vi "Analyse Board.vi"(8 "error in (no error)":errorcluster, 10 "GameBoard":u8[][](array[numeric]), 11 "CS++GoBangServer in":refnum<class "CS++GoBangServer.lvclass">) -> (0 "error out":errorcluster, 3 "CS++GoBangServer out":refnum<class "CS++GoBangServer.lvclass">)   [LabVIEW 2014, in "GoBang.lvlib" / "CS++GoBangServer.lvclass"]
uses:
  CS++GoBangServer.lvclass
  typdefs/GameState.ctl
  CS++GoBangServer.lvclass/CS++GoBangServer.ctl
  CSPP_Core/Classes/CS++ProcessVariables/ProcessVariable/PV.lvclass/PV.ctl
  CSPP_Core/Classes/CS++ProcessVariables/ProcessVariable/Write Data.vi
  GoBang.lvlib
  CSPP_Core/Classes/CS++ProcessVariables/ProcessVariable/PV.lvclass
  CSPP_Core/Classes/CS++ProcessVariables/PVConnection/PVConnection.lvclass
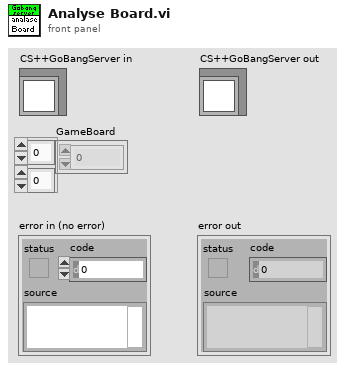
[diagram p1: front panel]
types:
  T1 = typedef "GoBang.lvlib/GameState.ctl" = enum16{"Waiting for opponent", "White to move", "Black to move", "Game over, white won", "Game over, black won"}
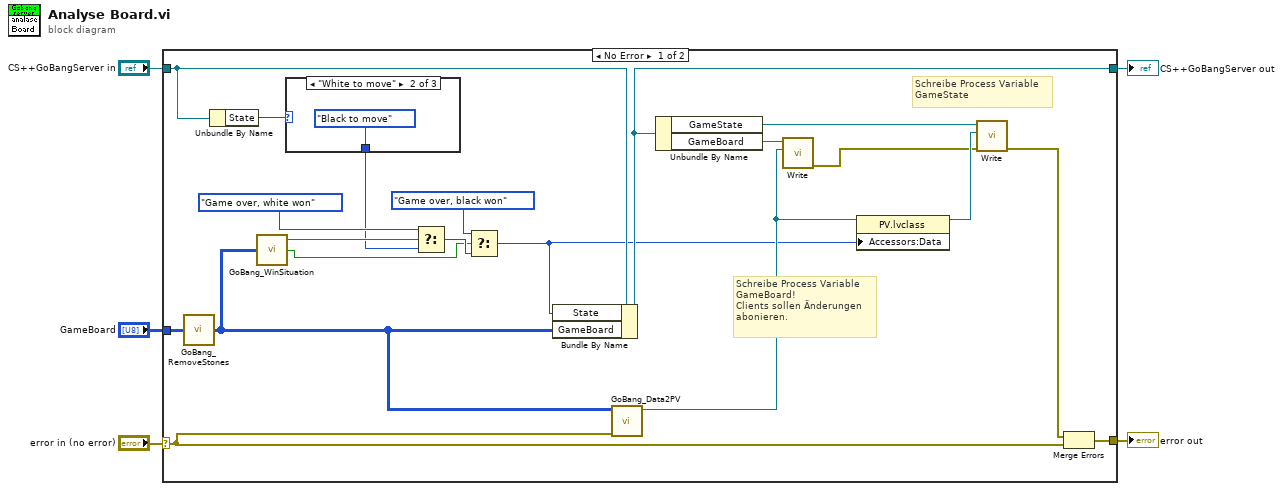
[diagram p0: block diagram]
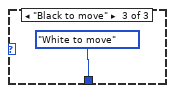
[diagram p3: hidden frame]
diagram:
  n1 = case shown="No Error" "error in (no error)" {
    selector: "error in (no error)" -> [w22 w30]
    tunnel: [w20 w30] -> w4
    tunnel: [w24 w29] -> w2
    tunnel: "CS++GoBangServer in" -> [w13 w29]
    tunnel: "GameBoard" -> [w25 _]
    frame No Error {
      # "Schreibe Process Variable \nGameState"
      # "Schreibe Process Variable \nGameBoard!\nClients sollen Änderungen\nabonieren."
      n2 = call "GoBang_RemoveStones.vi"("GameBoard in"=w25) -> ("GameBoard out"=w21:u8[][])
      n3 = Unbundle By Name(w13) -> ("State"=w9:T1)
      n4 = call "GoBang_WinSituation.vi"("GameBoard"=w21) -> ("White won"=w15:bool, "Black won"=w11:bool)  [unwired: 1 out]
      n5 = case shown="\"White to move\"" w9 {
        selector: w9 -> [w26 _ _]
        tunnel: [w26 GameState."Black to move" ("State") GameState."White to move" ("State")] -> w8
        frame "Waiting for opponent", Default {
        }
        frame "White to move" {
        }
        frame "Black to move" {
        }
      }
      n6 = Select(t=GameState."Game over, white won" ("State"), s=w15, f=w8) -> (s? t:f=w12:T1)
      n7 = Select(t=GameState."Game over, black won" ("State"), s=w11, f=w12) -> (s? t:f=w7:T1)
      n8 = Bundle By Name(cluster=w13, "State"=w7, "GameBoard"=w21) -> (w24:refnum<class "CS++GoBangServer.lvclass">)
      n9 = call "GoBang_Data2PV.vi"("error in (no error)"=w22, "Data in"=w21) -> ("PV out"=w18:refnum<class "PV.lvclass">)  [unwired: 9 in]
      n10 = Unbundle By Name(w24) -> ("GameState"=w19:refnum<class "PVConnection.lvclass">, "GameBoard"=w23:refnum<class "PVConnection.lvclass">)
      n11 = call "Write.vi"("PV"=w18, "PVConnection in"=w23) -> ("error out"=w6:errorcluster)  [unwired: 8 in, 1 out]
      n12 = property class="PV.lvclass"(reference=w18, "Accessors:Data"=w7) -> (reference out=w17:refnum<class "PV.lvclass">)  [unwired: 1 in, 1 out]
      n13 = call "Write.vi"("error in (no error)"=w6, "PV"=w17, "PVConnection in"=w19) -> ("error out"=w16:errorcluster)  [unwired: 7 in, 1 out]
      n14 = Merge Errors(w16, w22) -> (w20:errorcluster)
    }
    frame Error {
    }
  }
  "error out" <- w4
  "CS++GoBangServer out" <- w2
